vi "ATF-Do Index FGV.vi"(7 "State":enum16{"Write", "Read"}(ring)=enum."Read", 9 "Pumb index":i32[](array[numeric]), 11 "Storage index":i32[](array[numeric])) -> (1 "Pumb index 2":i32[](array[numeric]), 3 "Storage index":i32[](array[numeric]))   [LabVIEW 2022 SP3]
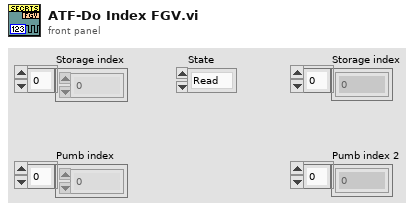
[diagram p1: front panel]
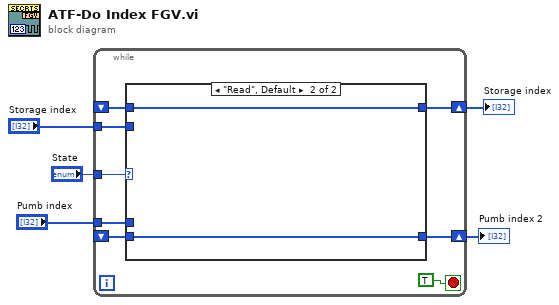
[diagram p0: block diagram]
diagram:
  n1 = while {
    tunnel: "State" -> [w12]
    shift-right: [w10] -> w3
    shift-left: _ -> [w11]
    tunnel: "Storage index" -> [w9]
    tunnel: "Pumb index" -> [w8]
    shift-right: [w7] -> w1
    shift-left: _ -> [w6]
    stop <- TRUE stop-if-true
    n2 = case shown="\"Read\", Default" w12 {
      tunnel: w11 -> [_ w17]
      tunnel: [w15 w17] -> w10
      tunnel: w9 -> [w15 _]
      tunnel: w8 -> [w14 _]
      tunnel: [w14 w16] -> w7
      tunnel: w6 -> [_ w16]
      frame "Write" {
      }
      frame "Read", Default {
      }
    }
  }
  "Storage index" <- w3
  "Pumb index 2" <- w1
